vi "Reference2miniscans.vi"(8 "error in (no error)":errorcluster) -> (0 "error out":errorcluster, 1 "Ref Zoom":dbl[](array[numeric]), 2 "miniScan_Coordinates":T1, 3 "miniScan Array":dbl[][](array[numeric]), 4 "Laser(V)":dbl[](array[numeric]), 5 "No of Miniscans":i32, 7 "No of Pixels":i32)   [LabVIEW 2020]
uses:
  Global Variables/General Globals.vi
panel:
  in  "XY(F)/Z(T)":bool=TRUE
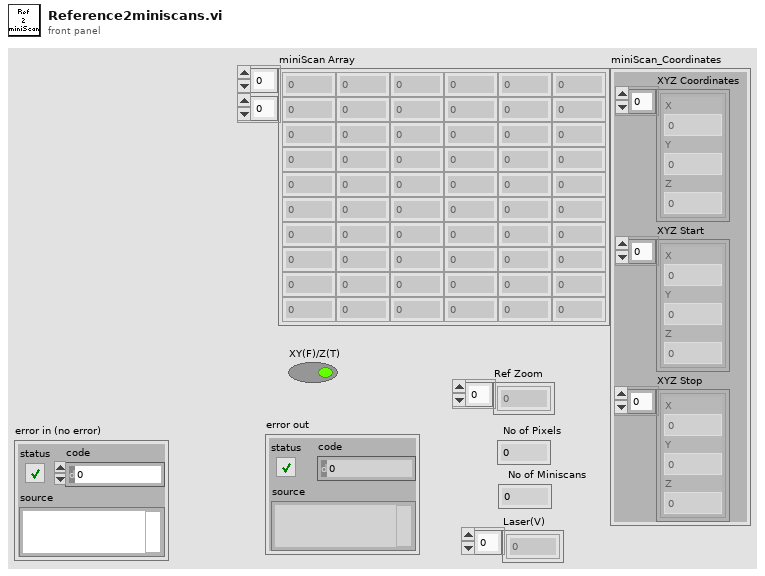
[diagram p1: front panel]
types:
  T1 = cluster{"XYZ Coordinates":cluster{"X":sgl, "Y":sgl, "Z":sgl}[], "XYZ Start":cluster{"X":dbl, "Y":dbl, "Z":dbl}[], "XYZ Stop":cluster{"X":dbl, "Y":dbl, "Z":dbl}[]}
  T2 = typedef "Reference_Globals.ctl" = cluster{"Refrence data path":path, "Reference Rectangle":i16[][], "AOL Z":dbl, "No of pixels in a miniscan ":i32[], "Threshold":i16[], "No of miniscans":i32[], "Full Frame Size":u16, "Reference Image":T3, "dwelltime":dbl, "Zoom":dbl, "Field of View":dbl, "Z Step":i8, "Z pixels":i32, "Z Lines":u8, "Z Ignore":u8, "Laser":u8, "Auto centering":bool}
  T3 = typedef "IMAQ Image.ctl" = refnum<image>
  T4 = typedef "Ref DAQ Param.ctl" = cluster{"Full Frame Size":u16, "Ref Field of View":sgl, "Ref Zoom":i8, "Ref_dwellTime":sgl, "Ref X-pixels-per-line(Npxr)":i16, "Ref Y-lines-per-image(Npyr)":i16, "Ref Z-lines-per-image":i16, "Ignore Z lines":i16, "Ref Scan Cycles":i32, "Ref threshold XY":u16, "Ref threshold Z":u16, "Ref average XY":u16, "Ref Average  Z":u16, "Proportional_scale":fxp<+,16,2>, "Integral_scale":fxp<+/-,16,12>, "Proportional_scale Z":fxp<+,16,2>, "Integral_scale Z":fxp<+/-,16,12>, "Diff_threshold":fxp<+,16,2>, "Diff_threshold _z":fxp<+,16,2>, "Sliding Average":bool, "Ref count reset enabled":bool, "Auto-centering":bool}
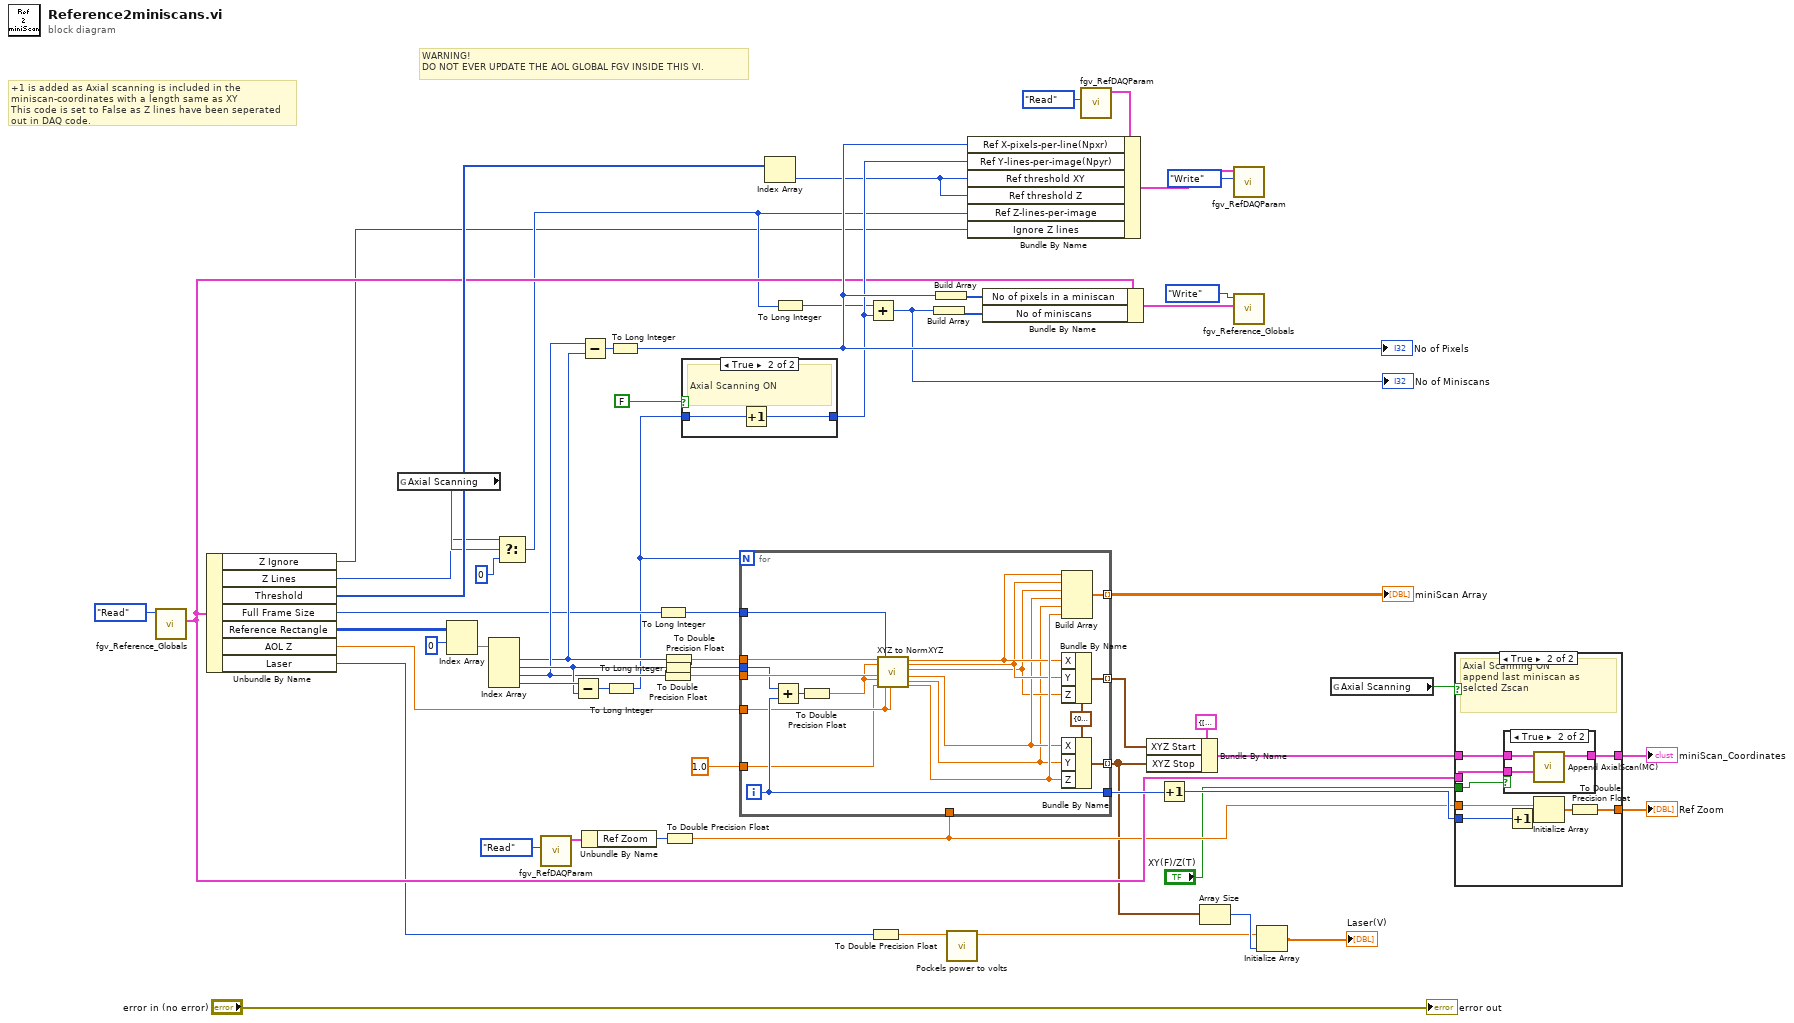
[diagram p0: block diagram]
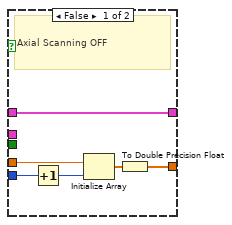
[diagram p3: hidden frame]
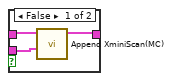
[diagram p4: hidden frame]
diagram:
  # "+1 is added as Axial scanning is included in the miniscan-coordinates with a length same as XY\nThis code is set to False as Z lines have been seperated out in DAQ code."
  # "WARNING!\nDO NOT EVER UPDATE THE AOL GLOBAL FGV INSIDE THIS VI."
  n1 = call "fgv_Reference_Globals.vi"("Function"=enum16{"Intialize", "Write", "Read", "Clear"}."Read") -> ("Reference Data"=w23:T2)  [unwired: 9 in, 1 out]
  n2 = Unbundle By Name(w23) -> ("Z Ignore"=w1:u8, "Z Lines"=w15:u8, "Threshold"=w38:i16[], "Full Frame Size"=w48:u16, "Reference Rectangle"=w49:i16[][], "AOL Z"=w29:dbl, "Laser"=w9:u8)
  n3 = global read "General Globals.vi" "Axial Scanning"() -> (w16:bool)
  n4 = Index Array(array=w49, index (row)=0) -> (element=w60:i16[])  [unwired: 1 in]
  n5 = Index Array(array=w60) -> (element #1=w51:i16, element #2=w58:i16, element #3=w53:i16, element #4=w59:i16)  [unwired: 4 in]
  n6 = Select(t=w15, s=w16, f=u8 0) -> (s? t:f=w3:u8)
  n7 = call "fgv_RefDAQParam.vi"("Function"=enum16{"Initialize", "Write", "Read"}."Read" ("Status")) -> ("RefDAQParam"=w33:T4)  [unwired: 9 in, 1 out]
  n8 = Subtract(x=w59, y=w58) -> (x-y=w54:i16)
  n9 = Subtract(x=w53, y=w51) -> (x-y=w52:i16)
  n10 = Unbundle By Name(w33) -> ("Ref Zoom"=w28:i8)
  n11 = To Long Integer(number=w54) -> (32bit integer=w24:i32)
  n12 = To Long Integer(number=w52) -> (32bit integer=w31:i32)
  "No of Pixels" <- w31
  n13 = To Long Integer(number=w48) -> (32bit integer=w35:i32)
  n14 = To Long Integer(number=w58) -> (32bit integer=w27:i32)
  n15 = To Double Precision Float(number=w53) -> (double precision float=w36:dbl)
  n16 = To Double Precision Float(number=w51) -> (double precision float=w37:dbl)
  n17 = To Double Precision Float(number=w28) -> (double precision float=w19:dbl)
  n18 = case shown="True" FALSE {
    tunnel: [w61 w63] -> w25
    tunnel: w24 -> [w61 w62]
    frame False {
      # "Axial Scanning OFF"
    }
    frame True {
      # "Axial Scanning ON"
      n19 = Increment(x=w62) -> (x+1=w63:i32)
    }
  }
  n20 = for {
    N: w24 -> [_]
    tunnel: w27 -> [w65]
    tunnel: w36 -> [w75]
    tunnel: w37 -> [w79]
    tunnel: [w82] -> w57 mode=indexing
    tunnel: w29 -> [w76]
    tunnel: [w81] -> w55 mode=indexing
    tunnel: [w80] -> w11 mode=indexing
    tunnel: w35 -> [w77]
    tunnel: [w78] -> w32
    tunnel: w19 -> [_]
    tunnel: 1.0 -> [w66]
    i -> [w78]
    w69 = cluster{"X":dbl, "Y":dbl, "Z":dbl} {"X"=0.0, "Y"=0.0, "Z"=0.0} ("XYZ")
    n21 = Add(x=w65, y=w78) -> (x+y=w74:i32)
    n22 = To Double Precision Float(number=w74) -> (double precision float=w72:dbl)
    n23 = call "XYZ to NormXYZ.vi"("X start"=w79, "Y start"=w72, "X stop"=w75, "Y stop"=w72, "Zoom (either ref or main zoom)"=w66, "FrameSize"=w77, "Z start"=w76, "Z stop"=w76) -> ("Norm X Start"=w71:dbl, "Norm Y Start"=w70:dbl, "Norm Z Start"=w67:dbl, "Norm X Stop"=w68:dbl, "Norm Y Stop"=w64:dbl, "Norm Z Stop"=w73:dbl)  [unwired: 6 in]
    n24 = Build Array(w71, w70, w67, w68, w64, w73) -> (w82:dbl[])
    n25 = Bundle By Name(cluster=w69, "X"=w71, "Y"=w70, "Z"=w67) -> (w81:cluster{"X":dbl, "Y":dbl, "Z":dbl})
    n26 = Bundle By Name(cluster=w69, "X"=w68, "Y"=w64, "Z"=w73) -> (w80:cluster{"X":dbl, "Y":dbl, "Z":dbl})
  }
  "miniScan Array" <- w57
  n27 = Index Array(array=w38) -> (element=w2:i16)  [unwired: 1 in]
  n28 = To Long Integer(number=w3) -> (32bit integer=w14:i32)
  n29 = Add(x=w14, y=w25) -> (x+y=w13:i32)
  "No of Miniscans" <- w13
  n30 = To Double Precision Float(number=w9) -> (double precision float=w6:dbl)
  n31 = Build Array(w13) -> (w43:i32[])
  n32 = Build Array(w31) -> (w44:i32[])
  n33 = call "Pockels power to volts.vi"("Pockels power (%)"=w6) -> ("Pockels control voltage (V)"=w8:dbl)  [unwired: 8 in, 2 out]
  n34 = Bundle By Name(cluster=w23, "No of pixels in a miniscan"=w44, "No of miniscans"=w43) -> (w45:T2)
  n35 = call "fgv_RefDAQParam.vi"("Function"=enum16{"Initialize", "Write", "Read"}."Read" ("Status")) -> ("RefDAQParam"=w39:T4)  [unwired: 9 in, 1 out]
  n36 = Bundle By Name(cluster=w39, "Ref X-pixels-per-line(Npxr)"=w31, "Ref Y-lines-per-image(Npyr)"=w25, "Ref threshold XY"=w2, "Ref threshold Z"=w2, "Ref Z-lines-per-image"=w3, "Ignore Z lines"=w1) -> (w30:T4)
  n37 = Bundle By Name(cluster=T1 {"XYZ Coordinates"=[], "XYZ Start"=[], "XYZ Stop"=[]} ("miniScan_Coordinates"), "XYZ Start"=w55, "XYZ Stop"=w11) -> (w26:T1)
  n38 = Increment(x=w32) -> (x+1=w20:i32)
  n39 = Array Size(array=w11) -> (size(s)=w10:i32)
  n40 = call "fgv_RefDAQParam.vi"("Function"=enum16{"Initialize", "Write", "Read"}."Write" ("Status"), "RefDAQParam in"=w30) -> ()  [unwired: 8 in, 2 out]
  n41 = call "fgv_Reference_Globals.vi"("Reference Data"=w45, "Function"=enum16{"Intialize", "Write", "Read", "Clear"}."Write") -> ()  [unwired: 8 in, 2 out]
  n42 = Initialize Array(w8, w10) -> (→"Laser(V)":dbl[])
  n43 = global read "General Globals.vi" "Axial Scanning"() -> (w4:bool)
  n44 = case shown="True" w4 {
    tunnel: [w88 w97] -> w22
    tunnel: w26 -> [w88 w96]
    tunnel: w23 -> [_ w95]
    tunnel: [w85 w93] -> w21
    tunnel: w20 -> [w83 w92]
    tunnel: w19 -> [w84 w90]
    tunnel: "XY(F)/Z(T)" -> [_ w89]
    frame False {
      # "Axial Scanning OFF"
      n45 = Increment(x=w83) -> (x+1=w86:i32)
      n46 = Initialize Array(w84, w86) -> (w87:dbl[])
      n47 = To Double Precision Float(number=w87) -> (double precision float=w85:dbl[])
    }
    frame True {
      # "Axial Scanning ON\nappend last miniscan as selcted Zscan"
      n48 = case shown="True" w89 {
        tunnel: [w99 w103] -> w97
        tunnel: w96 -> [w100 w102]
        tunnel: w95 -> [w98 w101]
        frame False {
          n49 = call "Append XminiScan(MC).vi"("Reference Data"=w98, "miniScan_Coordinates"=w100) -> ("miniScan_Coordinates"=w99:T1)  [unwired: 9 in]
        }
        frame True {
          n50 = call "Append AxialScan(MC).vi"("Reference Data"=w101, "miniScan_Coordinates"=w102) -> ("miniScan_Coordinates"=w103:T1)  [unwired: 9 in]
        }
      }
      n51 = Increment(x=w92) -> (x+1=w91:i32)
      n52 = Initialize Array(w90, w91) -> (w94:dbl[])
      n53 = To Double Precision Float(number=w94) -> (double precision float=w93:dbl[])
    }
  }
  "miniScan_Coordinates" <- w22
  "Ref Zoom" <- w21
  "error out" <- "error in (no error)"
